vi "sample6(Velo&Acc PRO).vi"() -> ()   [LabVIEW 2020]
panel:
  out "Error Flag":T1
  out "err":errorcluster caption="エラー出力" {"code" format="%04x"}
  in  "TorqueEnable":bool
  in  "GOAL ACCELERATION":i32(knob) scale=0.0..400.0
  in  "GOAL VELOCITY":i32(knob) scale=0.0..8000.0
  in  "OffsetTime":u32=500
  out "PRESENT POSITION":i32
  in  "ID":u8=1 max=253
  in  "Baudrate":u32=57600
  in  "COM":refnum<visa-resource-name> caption="COMポート"
  in  "STOP":bool
  in  "GOAL POSITION":i32(knob) scale=100000.0..-100000.0
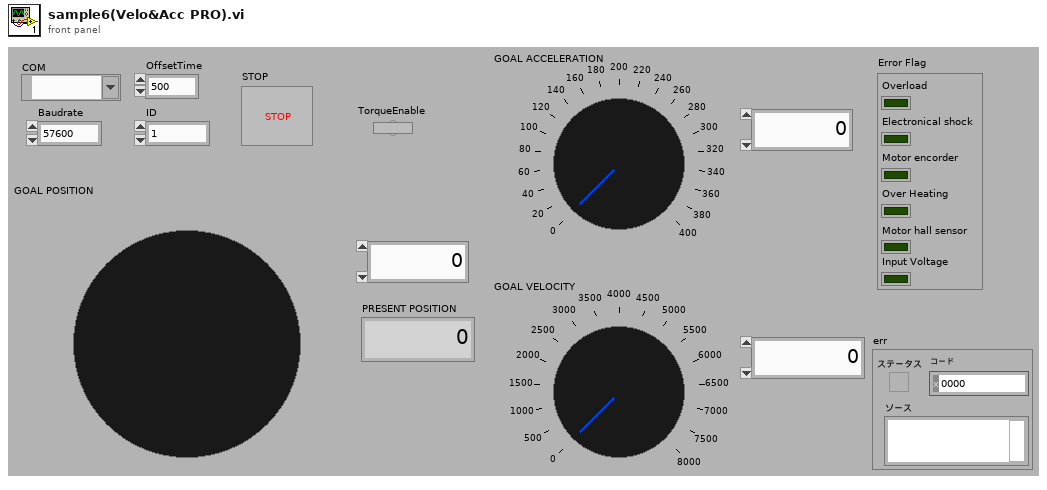
[diagram p1: front panel]
types:
  T1 = cluster{"Input Voltage":bool, "Motor hall sensor":bool, "Over Heating":bool, "Motor encorder":bool, "Electronical shock":bool, "Overload":bool}
  T2 = cluster{"Boolean array[0]":bool, "Boolean array[1]":bool, "Boolean array[2]":bool, "Boolean array[3]":bool, "Boolean array[4]":bool, "Boolean array[5]":bool}
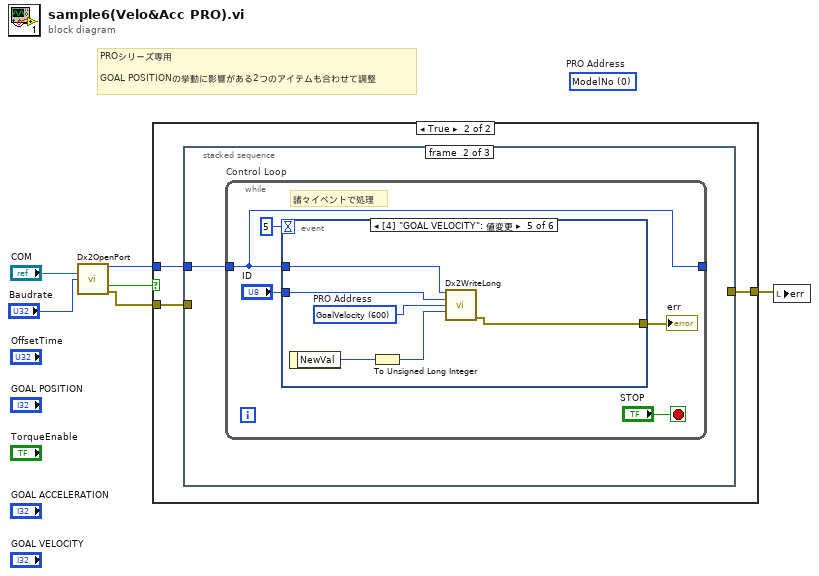
[diagram p0: block diagram]
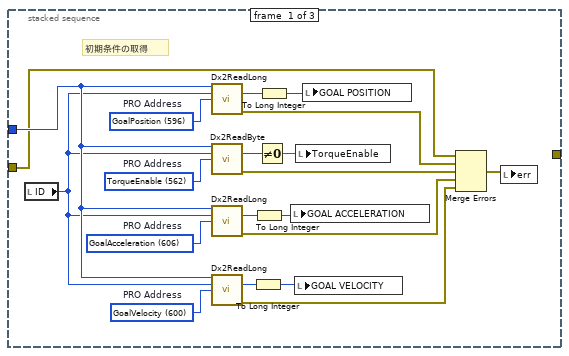
[diagram p3: hidden frame]
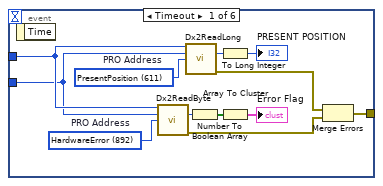
[diagram p4: hidden frame]
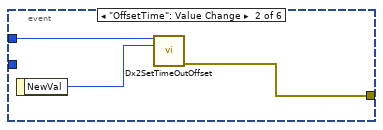
[diagram p5: hidden frame]
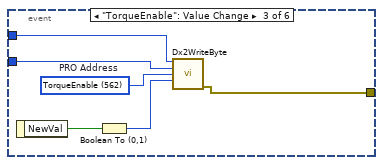
[diagram p6: hidden frame]
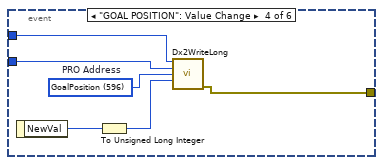
[diagram p7: hidden frame]
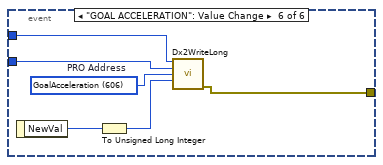
[diagram p8: hidden frame]
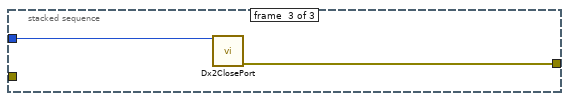
[diagram p9: hidden frame]
diagram:
  (unwired) u16 0 items=["ModelNo"=0, "ModelInfo"=2, "VersionOfFirmware"=6, "ID"=7, "Baudrate"=8, "ReturnDelayTime"=9, "OperationMode"=11, "HormingOffset"=13, "MovingThreshold"=17, "TemperatureLimit"=21, "MaxVoltageLimit"=22, "MinVoltageLimit"=24, "AccelerationLimit"=26, "TorqueLimit"=30, "VoltageLimit"=32, "MaxPositionLimit"=36, "MinPositionLimit"=40, "ExternalPortMode1"=44, "ExternalPortMode2"=45, "ExternalPortMode3"=46, "ExternalPortMode4"=47, "Shutdown"=48, "TorqueEnable"=562, "LED_Red"=563, "LED_Green"=564, "LED_Blue"=565, "VelocityIGain"=586, "VelocityPGain"=588, "PositionPGain"=594, "GoalPosition"=596, "GoalVelocity"=600, "GoalTorque"=604, "GoalAcceleration"=606, "Moving"=610, "PresentPosition"=611, "PresentVelocity"=615, "PresentCurrent"=621, "PresentInputVoltage"=623, "PresentTemperature"=625, "ExternalPortData1"=626, "ExternalPortData2"=628, "ExternalPortData3"=630, "ExternalPortData4"=632, "RegistedInstruction"=890, "StatusReturnLevel"=891, "HardwareError"=892]  # PRO Address
  # "PROシリーズ専用\n\nGOAL POSITIONの挙動に影響がある2つのアイテムも合わせて調整"
  n1 = call "Dx2OpenPort.vi"("port"="COM", "baudrate"="Baudrate") -> ("dvid"=w4:u32, "成功"=w3:bool, "エラー出力"=w2:errorcluster)  [unwired: 11 in]
  n2 = case shown="TRUE" w3 {
    tunnel: w4 -> [_ w10]
    tunnel: w2 -> [w7 w9]
    tunnel: [w7 w8] -> w1
    frame False {
    }
    frame True {
      n3 = stacked-sequence {
        tunnel: w10 -> [w24 w31 w77]
        tunnel: [_ _ w76] -> w8
        tunnel: w9 -> [w17 _ _]
        frame #0 {
          w11 = u16 600 items=["ModelNo"=0, "ModelInfo"=2, "VersionOfFirmware"=6, "ID"=7, "Baudrate"=8, "ReturnDelayTime"=9, "OperationMode"=11, "HormingOffset"=13, "MovingThreshold"=17, "TemperatureLimit"=21, "MaxVoltageLimit"=22, "MinVoltageLimit"=24, "AccelerationLimit"=26, "TorqueLimit"=30, "VoltageLimit"=32, "MaxPositionLimit"=36, "MinPositionLimit"=40, "ExternalPortMode1"=44, "ExternalPortMode2"=45, "ExternalPortMode3"=46, "ExternalPortMode4"=47, "Shutdown"=48, "TorqueEnable"=562, "LED_Red"=563, "LED_Green"=564, "LED_Blue"=565, "VelocityIGain"=586, "VelocityPGain"=588, "PositionPGain"=594, "GoalPosition"=596, "GoalVelocity"=600, "GoalTorque"=604, "GoalAcceleration"=606, "Moving"=610, "PresentPosition"=611, "PresentVelocity"=615, "PresentCurrent"=621, "PresentInputVoltage"=623, "PresentTemperature"=625, "ExternalPortData1"=626, "ExternalPortData2"=628, "ExternalPortData3"=630, "ExternalPortData4"=632, "RegistedInstruction"=890, "StatusReturnLevel"=891, "HardwareError"=892]  # PRO Address
          w12 = u16 606 items=["ModelNo"=0, "ModelInfo"=2, "VersionOfFirmware"=6, "ID"=7, "Baudrate"=8, "ReturnDelayTime"=9, "OperationMode"=11, "HormingOffset"=13, "MovingThreshold"=17, "TemperatureLimit"=21, "MaxVoltageLimit"=22, "MinVoltageLimit"=24, "AccelerationLimit"=26, "TorqueLimit"=30, "VoltageLimit"=32, "MaxPositionLimit"=36, "MinPositionLimit"=40, "ExternalPortMode1"=44, "ExternalPortMode2"=45, "ExternalPortMode3"=46, "ExternalPortMode4"=47, "Shutdown"=48, "TorqueEnable"=562, "LED_Red"=563, "LED_Green"=564, "LED_Blue"=565, "VelocityIGain"=586, "VelocityPGain"=588, "PositionPGain"=594, "GoalPosition"=596, "GoalVelocity"=600, "GoalTorque"=604, "GoalAcceleration"=606, "Moving"=610, "PresentPosition"=611, "PresentVelocity"=615, "PresentCurrent"=621, "PresentInputVoltage"=623, "PresentTemperature"=625, "ExternalPortData1"=626, "ExternalPortData2"=628, "ExternalPortData3"=630, "ExternalPortData4"=632, "RegistedInstruction"=890, "StatusReturnLevel"=891, "HardwareError"=892]  # PRO Address
          w13 = u16 562 items=["ModelNo"=0, "ModelInfo"=2, "VersionOfFirmware"=6, "ID"=7, "Baudrate"=8, "ReturnDelayTime"=9, "OperationMode"=11, "HormingOffset"=13, "MovingThreshold"=17, "TemperatureLimit"=21, "MaxVoltageLimit"=22, "MinVoltageLimit"=24, "AccelerationLimit"=26, "TorqueLimit"=30, "VoltageLimit"=32, "MaxPositionLimit"=36, "MinPositionLimit"=40, "ExternalPortMode1"=44, "ExternalPortMode2"=45, "ExternalPortMode3"=46, "ExternalPortMode4"=47, "Shutdown"=48, "TorqueEnable"=562, "LED_Red"=563, "LED_Green"=564, "LED_Blue"=565, "VelocityIGain"=586, "VelocityPGain"=588, "PositionPGain"=594, "GoalPosition"=596, "GoalVelocity"=600, "GoalTorque"=604, "GoalAcceleration"=606, "Moving"=610, "PresentPosition"=611, "PresentVelocity"=615, "PresentCurrent"=621, "PresentInputVoltage"=623, "PresentTemperature"=625, "ExternalPortData1"=626, "ExternalPortData2"=628, "ExternalPortData3"=630, "ExternalPortData4"=632, "RegistedInstruction"=890, "StatusReturnLevel"=891, "HardwareError"=892]  # PRO Address
          w14 = u16 596 items=["ModelNo"=0, "ModelInfo"=2, "VersionOfFirmware"=6, "ID"=7, "Baudrate"=8, "ReturnDelayTime"=9, "OperationMode"=11, "HormingOffset"=13, "MovingThreshold"=17, "TemperatureLimit"=21, "MaxVoltageLimit"=22, "MinVoltageLimit"=24, "AccelerationLimit"=26, "TorqueLimit"=30, "VoltageLimit"=32, "MaxPositionLimit"=36, "MinPositionLimit"=40, "ExternalPortMode1"=44, "ExternalPortMode2"=45, "ExternalPortMode3"=46, "ExternalPortMode4"=47, "Shutdown"=48, "TorqueEnable"=562, "LED_Red"=563, "LED_Green"=564, "LED_Blue"=565, "VelocityIGain"=586, "VelocityPGain"=588, "PositionPGain"=594, "GoalPosition"=596, "GoalVelocity"=600, "GoalTorque"=604, "GoalAcceleration"=606, "Moving"=610, "PresentPosition"=611, "PresentVelocity"=615, "PresentCurrent"=621, "PresentInputVoltage"=623, "PresentTemperature"=625, "ExternalPortData1"=626, "ExternalPortData2"=628, "ExternalPortData3"=630, "ExternalPortData4"=632, "RegistedInstruction"=890, "StatusReturnLevel"=891, "HardwareError"=892]  # PRO Address
          # "初期条件の取得"
          n4 = local read "ID"() -> (w23:u8)
          n5 = call "Dx2ReadLong.vi"("dvid in"=w24, "id"=w23, "address"=w14) -> ("data out"=w16:u32, "エラー出力"=w22:errorcluster)  [unwired: 9 in, 2 out]
          n6 = call "Dx2ReadByte.vi"("dvid in"=w24, "id"=w23, "address"=w13) -> ("data out"=w30:u8, "エラー出力"=w21:errorcluster)  [unwired: 9 in, 2 out]
          n7 = call "Dx2ReadLong.vi"("dvid in"=w24, "id"=w23, "address"=w12) -> ("data out"=w27:u32, "エラー出力"=w20:errorcluster)  [unwired: 9 in, 2 out]
          n8 = call "Dx2ReadLong.vi"("dvid in"=w24, "id"=w23, "address"=w11) -> ("data out"=w26:u32, "エラー出力"=w19:errorcluster)  [unwired: 9 in, 2 out]
          n9 = To Long Integer(number=w26) -> (32bit integer=w25:i32)
          n10 = To Long Integer(number=w27) -> (32bit integer=w28:i32)
          n11 = Not Equal To 0?(x=w30) -> (x != 0?=w29:bool)
          n12 = To Long Integer(number=w16) -> (32bit integer=w15:i32)
          n13 = local write "GOAL ACCELERATION"(w28) -> ()
          n14 = local write "GOAL VELOCITY"(w25) -> ()
          n15 = local write "TorqueEnable"(w29) -> ()
          n16 = local write "GOAL POSITION"(w15) -> ()
          n17 = Merge Errors(w17, w22, w21, w20, w19) -> (w18:errorcluster)
          n18 = local write "err"(w18) -> ()
        }
        frame #1 {
          n19 = while "Control Loop" {
            tunnel: w31 -> [w34]
            tunnel: [w34] -> _
            stop <- "STOP" stop-if-true
            # "諸々イベントで処理"
            n20 = event shown="[4] \"GOAL VELOCITY\": 値変更" {
              selector: _ -> [_ _ _ _ _ _]
              dyn-events: _ -> [_ _ _ _ _ _]
              timeout: 5 -> [_ _ _ _ _ _]
              tunnel: "ID" -> [w42 _ w57 w63 w69 w75]
              tunnel: w34 -> [w43 w50 w56 w62 w68 w74]
              tunnel: [w37 w49 w53 w59 w65 w71] -> w33
              event Timeout {
                w40 = u16 892 items=["ModelNo"=0, "ModelInfo"=2, "VersionOfFirmware"=6, "ID"=7, "Baudrate"=8, "ReturnDelayTime"=9, "OperationMode"=11, "HormingOffset"=13, "MovingThreshold"=17, "TemperatureLimit"=21, "MaxVoltageLimit"=22, "MinVoltageLimit"=24, "AccelerationLimit"=26, "TorqueLimit"=30, "VoltageLimit"=32, "MaxPositionLimit"=36, "MinPositionLimit"=40, "ExternalPortMode1"=44, "ExternalPortMode2"=45, "ExternalPortMode3"=46, "ExternalPortMode4"=47, "Shutdown"=48, "TorqueEnable"=562, "LED_Red"=563, "LED_Green"=564, "LED_Blue"=565, "VelocityIGain"=586, "VelocityPGain"=588, "PositionPGain"=594, "GoalPosition"=596, "GoalVelocity"=600, "GoalTorque"=604, "GoalAcceleration"=606, "Moving"=610, "PresentPosition"=611, "PresentVelocity"=615, "PresentCurrent"=621, "PresentInputVoltage"=623, "PresentTemperature"=625, "ExternalPortData1"=626, "ExternalPortData2"=628, "ExternalPortData3"=630, "ExternalPortData4"=632, "RegistedInstruction"=890, "StatusReturnLevel"=891, "HardwareError"=892]  # PRO Address
                w41 = u16 611 items=["ModelNo"=0, "ModelInfo"=2, "VersionOfFirmware"=6, "ID"=7, "Baudrate"=8, "ReturnDelayTime"=9, "OperationMode"=11, "HormingOffset"=13, "MovingThreshold"=17, "TemperatureLimit"=21, "MaxVoltageLimit"=22, "MinVoltageLimit"=24, "AccelerationLimit"=26, "TorqueLimit"=30, "VoltageLimit"=32, "MaxPositionLimit"=36, "MinPositionLimit"=40, "ExternalPortMode1"=44, "ExternalPortMode2"=45, "ExternalPortMode3"=46, "ExternalPortMode4"=47, "Shutdown"=48, "TorqueEnable"=562, "LED_Red"=563, "LED_Green"=564, "LED_Blue"=565, "VelocityIGain"=586, "VelocityPGain"=588, "PositionPGain"=594, "GoalPosition"=596, "GoalVelocity"=600, "GoalTorque"=604, "GoalAcceleration"=606, "Moving"=610, "PresentPosition"=611, "PresentVelocity"=615, "PresentCurrent"=621, "PresentInputVoltage"=623, "PresentTemperature"=625, "ExternalPortData1"=626, "ExternalPortData2"=628, "ExternalPortData3"=630, "ExternalPortData4"=632, "RegistedInstruction"=890, "StatusReturnLevel"=891, "HardwareError"=892]  # PRO Address
                n21 = event-data() -> ()  [unwired: 1 in, 1 out]
                n22 = call "Dx2ReadByte.vi"("dvid in"=w43, "id"=w42, "address"=w40) -> ("data out"=w45:u8, "エラー出力"=w38:errorcluster)  [unwired: 9 in, 2 out]
                n23 = call "Dx2ReadLong.vi"("dvid in"=w43, "id"=w42, "address"=w41) -> ("data out"=w47:u32, "エラー出力"=w39:errorcluster)  [unwired: 9 in, 2 out]
                n24 = Number To Boolean Array(number=w45) -> (Boolean array=w46:bool[])
                n25 = To Long Integer(number=w47) -> (32bit integer=→"PRESENT POSITION":i32)
                n26 = Array To Cluster(array=w46) -> (cluster=→"Error Flag":T2)
                n27 = Merge Errors(w39, w38) -> (w37:errorcluster)
              }
              event "OffsetTime": Value Change {
                n28 = event-data() -> ("NewVal"=w51:u32)  [unwired: 1 in]
                n29 = call "Dx2SetTimeOutOffset.vi"("dvid in"=w50, "OffsetTime"=w51) -> ("エラー出力"=w49:errorcluster)  [unwired: 12 in, 1 out]
              }
              event "TorqueEnable": Value Change {
                w52 = u16 562 items=["ModelNo"=0, "ModelInfo"=2, "VersionOfFirmware"=6, "ID"=7, "Baudrate"=8, "ReturnDelayTime"=9, "OperationMode"=11, "HormingOffset"=13, "MovingThreshold"=17, "TemperatureLimit"=21, "MaxVoltageLimit"=22, "MinVoltageLimit"=24, "AccelerationLimit"=26, "TorqueLimit"=30, "VoltageLimit"=32, "MaxPositionLimit"=36, "MinPositionLimit"=40, "ExternalPortMode1"=44, "ExternalPortMode2"=45, "ExternalPortMode3"=46, "ExternalPortMode4"=47, "Shutdown"=48, "TorqueEnable"=562, "LED_Red"=563, "LED_Green"=564, "LED_Blue"=565, "VelocityIGain"=586, "VelocityPGain"=588, "PositionPGain"=594, "GoalPosition"=596, "GoalVelocity"=600, "GoalTorque"=604, "GoalAcceleration"=606, "Moving"=610, "PresentPosition"=611, "PresentVelocity"=615, "PresentCurrent"=621, "PresentInputVoltage"=623, "PresentTemperature"=625, "ExternalPortData1"=626, "ExternalPortData2"=628, "ExternalPortData3"=630, "ExternalPortData4"=632, "RegistedInstruction"=890, "StatusReturnLevel"=891, "HardwareError"=892]  # PRO Address
                n30 = event-data() -> ("NewVal"=w55:bool)  [unwired: 1 in]
                n31 = Boolean To (0,1)(Boolean=w55) -> (0, 1=w54:i16)
                n32 = call "Dx2WriteByte.vi"("dvid in"=w56, "id"=w57, "address"=w52, "data in"=w54) -> ("エラー出力"=w53:errorcluster)  [unwired: 9 in, 2 out]
              }
              event "GOAL POSITION": Value Change {
                w58 = u16 596 items=["ModelNo"=0, "ModelInfo"=2, "VersionOfFirmware"=6, "ID"=7, "Baudrate"=8, "ReturnDelayTime"=9, "OperationMode"=11, "HormingOffset"=13, "MovingThreshold"=17, "TemperatureLimit"=21, "MaxVoltageLimit"=22, "MinVoltageLimit"=24, "AccelerationLimit"=26, "TorqueLimit"=30, "VoltageLimit"=32, "MaxPositionLimit"=36, "MinPositionLimit"=40, "ExternalPortMode1"=44, "ExternalPortMode2"=45, "ExternalPortMode3"=46, "ExternalPortMode4"=47, "Shutdown"=48, "TorqueEnable"=562, "LED_Red"=563, "LED_Green"=564, "LED_Blue"=565, "VelocityIGain"=586, "VelocityPGain"=588, "PositionPGain"=594, "GoalPosition"=596, "GoalVelocity"=600, "GoalTorque"=604, "GoalAcceleration"=606, "Moving"=610, "PresentPosition"=611, "PresentVelocity"=615, "PresentCurrent"=621, "PresentInputVoltage"=623, "PresentTemperature"=625, "ExternalPortData1"=626, "ExternalPortData2"=628, "ExternalPortData3"=630, "ExternalPortData4"=632, "RegistedInstruction"=890, "StatusReturnLevel"=891, "HardwareError"=892]  # PRO Address
                n33 = event-data() -> ("NewVal"=w61:i32)  [unwired: 1 in]
                n34 = To Unsigned Long Integer(number=w61) -> (unsigned 32bit integer=w60:u32)
                n35 = call "Dx2WriteLong.vi"("dvid in"=w62, "id"=w63, "address"=w58, "data in"=w60) -> ("エラー出力"=w59:errorcluster)  [unwired: 9 in, 2 out]
              }
              event "GOAL VELOCITY": Value Change {
                w64 = u16 600 items=["ModelNo"=0, "ModelInfo"=2, "VersionOfFirmware"=6, "ID"=7, "Baudrate"=8, "ReturnDelayTime"=9, "OperationMode"=11, "HormingOffset"=13, "MovingThreshold"=17, "TemperatureLimit"=21, "MaxVoltageLimit"=22, "MinVoltageLimit"=24, "AccelerationLimit"=26, "TorqueLimit"=30, "VoltageLimit"=32, "MaxPositionLimit"=36, "MinPositionLimit"=40, "ExternalPortMode1"=44, "ExternalPortMode2"=45, "ExternalPortMode3"=46, "ExternalPortMode4"=47, "Shutdown"=48, "TorqueEnable"=562, "LED_Red"=563, "LED_Green"=564, "LED_Blue"=565, "VelocityIGain"=586, "VelocityPGain"=588, "PositionPGain"=594, "GoalPosition"=596, "GoalVelocity"=600, "GoalTorque"=604, "GoalAcceleration"=606, "Moving"=610, "PresentPosition"=611, "PresentVelocity"=615, "PresentCurrent"=621, "PresentInputVoltage"=623, "PresentTemperature"=625, "ExternalPortData1"=626, "ExternalPortData2"=628, "ExternalPortData3"=630, "ExternalPortData4"=632, "RegistedInstruction"=890, "StatusReturnLevel"=891, "HardwareError"=892]  # PRO Address
                n36 = event-data() -> ("NewVal"=w67:i32)  [unwired: 1 in]
                n37 = To Unsigned Long Integer(number=w67) -> (unsigned 32bit integer=w66:u32)
                n38 = call "Dx2WriteLong.vi"("dvid in"=w68, "id"=w69, "address"=w64, "data in"=w66) -> ("エラー出力"=w65:errorcluster)  [unwired: 9 in, 2 out]
              }
              event "GOAL ACCELERATION": Value Change {
                w70 = u16 606 items=["ModelNo"=0, "ModelInfo"=2, "VersionOfFirmware"=6, "ID"=7, "Baudrate"=8, "ReturnDelayTime"=9, "OperationMode"=11, "HormingOffset"=13, "MovingThreshold"=17, "TemperatureLimit"=21, "MaxVoltageLimit"=22, "MinVoltageLimit"=24, "AccelerationLimit"=26, "TorqueLimit"=30, "VoltageLimit"=32, "MaxPositionLimit"=36, "MinPositionLimit"=40, "ExternalPortMode1"=44, "ExternalPortMode2"=45, "ExternalPortMode3"=46, "ExternalPortMode4"=47, "Shutdown"=48, "TorqueEnable"=562, "LED_Red"=563, "LED_Green"=564, "LED_Blue"=565, "VelocityIGain"=586, "VelocityPGain"=588, "PositionPGain"=594, "GoalPosition"=596, "GoalVelocity"=600, "GoalTorque"=604, "GoalAcceleration"=606, "Moving"=610, "PresentPosition"=611, "PresentVelocity"=615, "PresentCurrent"=621, "PresentInputVoltage"=623, "PresentTemperature"=625, "ExternalPortData1"=626, "ExternalPortData2"=628, "ExternalPortData3"=630, "ExternalPortData4"=632, "RegistedInstruction"=890, "StatusReturnLevel"=891, "HardwareError"=892]  # PRO Address
                n39 = event-data() -> ("NewVal"=w73:i32)  [unwired: 1 in]
                n40 = To Unsigned Long Integer(number=w73) -> (unsigned 32bit integer=w72:u32)
                n41 = call "Dx2WriteLong.vi"("dvid in"=w74, "id"=w75, "address"=w70, "data in"=w72) -> ("エラー出力"=w71:errorcluster)  [unwired: 9 in, 2 out]
              }
            }
            "err" <- w33
          }
        }
        frame #2 {
          n42 = call "Dx2ClosePort.vi"("dvid"=w77) -> ("エラー出力"=w76:errorcluster)  [unwired: 13 in, 1 out]
        }
      }
    }
  }
  n43 = local write "err"(w1) -> ()
